vi "Calculate_Servo_Spin.vi"(6 "RightJoyStick X":dbl(slide) scale=-1.0..1.0, 8 "buttons.leftGrip":dbl=1e-06, 9 "buttons.rightGrip":dbl=1e-06, 10 "y":dbl, 11 "x":dbl) -> (0 "r scaled":dbl=0.007642847767684503, 1 "M3":dbl=0.007642847767684503, 2 "M2":dbl=0.007642847767684503, 3 "M1":dbl=0.007642847767684503)   [LabVIEW 2017]
panel:
  out "buttons.leftGrip (Not yet used)":dbl=1e-06
  out "max value":dbl=0.007516748932651743
  out "r":dbl=0.007642847767684503
  out "Theta3":dbl=220.4223221640822
  out "Theta2":dbl=100.4223221640822
  out "Theta1":dbl=-19.577677835917797
  out "Phi":dbl=109.5776778359178
  in  "alpha3":dbl=330.0
  in  "alpha2":dbl=210.0
  in  "alpha1":dbl=90.0
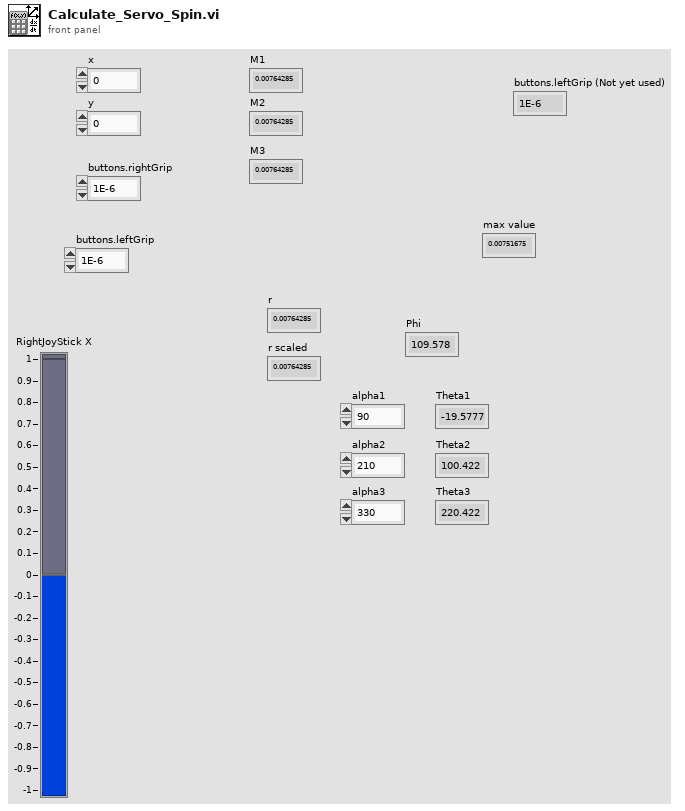
[diagram p1: front panel]
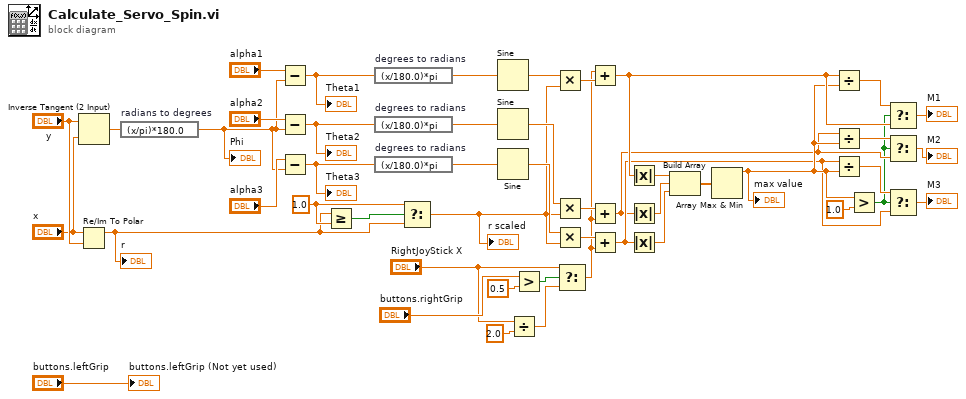
[diagram p0: block diagram]
diagram:
  w32 = 1.0 ("t")
  n1 = Inverse Tangent (2 Input)(1:"x", 2:"y") -> (0:w47:dbl)
  n2 = Re/Im To Polar(2:"y", 3:"x") -> (1:w6:dbl)  [unwired: 1 out]
  "r" <- w6
  n3 = expression code="(x/pi)*180.0" "radians to degrees"(w47) -> (w44:dbl)
  "Phi" <- w44
  n4 = Subtract(x="alpha1", y=w44) -> (x-y=w41:dbl)
  "Theta1" <- w41
  n5 = Subtract(x="alpha2", y=w44) -> (x-y=w43:dbl)
  "Theta2" <- w43
  n6 = Subtract(x="alpha3", y=w44) -> (x-y=w42:dbl)
  "Theta3" <- w42
  n7 = Greater Or Equal?(x=w6, y=w32) -> (x >= y?=w33:bool)
  n8 = expression code="(x/180.0)*pi" "degrees to radians"(w41) -> (w39:dbl)
  n9 = expression code="(x/180.0)*pi" "degrees to radians"(w43) -> (w37:dbl)
  n10 = expression code="(x/180.0)*pi" "degrees to radians"(w42) -> (w35:dbl)
  n11 = Select(t=w32, s=w33, f=w6) -> (s? t:f=w34:dbl)
  "r scaled" <- w34
  n12 = Sine(x=w39) -> (sin(x)=w40:dbl)
  n13 = Sine(x=w37) -> (sin(x)=w38:dbl)
  n14 = Sine(x=w35) -> (sin(x)=w36:dbl)
  n15 = Divide(x="RightJoyStick X", y=2.0) -> (x/y=w15:dbl)
  n16 = Greater?(x="buttons.rightGrip", y=0.5) -> (0:w14:bool)
  n17 = Multiply(x=w40, y=w34) -> (x*y=w29:dbl)
  n18 = Multiply(x=w38, y=w34) -> (x*y=w28:dbl)
  n19 = Multiply(x=w36, y=w34) -> (x*y=w27:dbl)
  n20 = Select(t="RightJoyStick X", s=w14, f=w15) -> (s? t:f=w12:dbl)
  n21 = Add(x=w12, y=w29) -> (x+y=w21:dbl)
  n22 = Add(x=w28, y=w12) -> (x+y=w16:dbl)
  n23 = Add(x=w27, y=w12) -> (x+y=w17:dbl)
  n24 = Absolute Value(x=w21) -> (abs(x)=w25:dbl)
  n25 = Absolute Value(x=w16) -> (abs(x)=w24:dbl)
  n26 = Absolute Value(x=w17) -> (abs(x)=w23:dbl)
  n27 = Build Array(w25, w24, w23) -> (w26:dbl[])
  n28 = Array Max & Min(array=w26) -> (max value=w18:dbl)  [unwired: 3 out]
  "max value" <- w18
  n29 = Divide(x=w21, y=w18) -> (x/y=w7:dbl)
  n30 = Divide(x=w16, y=w18) -> (x/y=w19:dbl)
  n31 = Divide(x=w17, y=w18) -> (x/y=w20:dbl)
  n32 = Greater?(x=w18, y=1.0) -> (0:w8:bool)
  n33 = Select(t=w7, s=w8, f=w21) -> (s? t:f=→"M1":dbl)
  n34 = Select(t=w19, s=w8, f=w16) -> (s? t:f=→"M2":dbl)
  n35 = Select(t=w20, s=w8, f=w17) -> (s? t:f=→"M3":dbl)
  "buttons.leftGrip (Not yet used)" <- "buttons.leftGrip"
